vi "script user process vi.vi"(8 "error in":errorcluster, 10 "runtime class path in":path, 11 "Application in":refnum<vi>) -> (0 "error out":errorcluster)   [LabVIEW 2013]
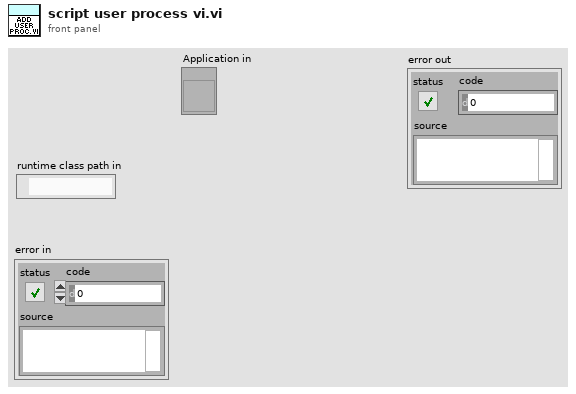
[diagram p1: front panel]
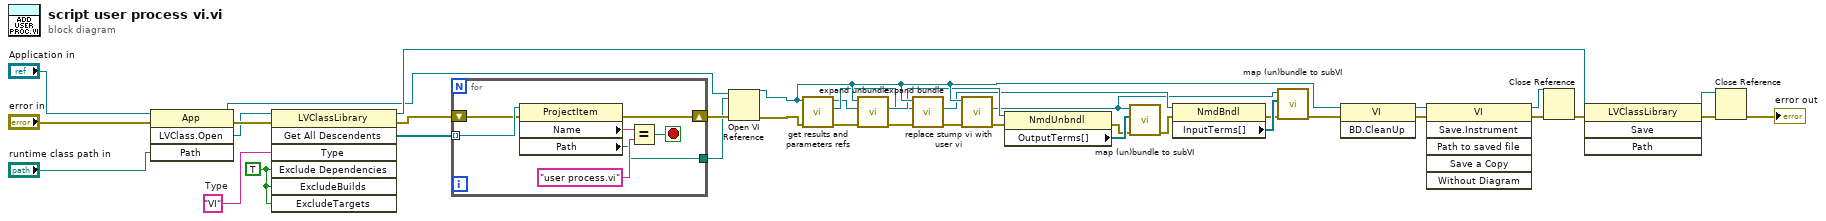
[diagram p0: block diagram]
diagram:
  w37 = TRUE
  w36 = "VI"  # Type
  n1 = invoke class="App" method="LVClass.Open"(reference="Application in", error in="error in", "Path"="runtime class path in") -> (reference out=w15:refnum<vi>, error out=w38:errorcluster, "LVClass.Open"=w16:refnum<vi>)  [unwired: 1 in, 1 out]
  n2 = invoke class="LVClassLibrary" method="Get All Descendents"(reference=w16, error in=w38, "Type"=w36, "Exclude Dependencies"=w37, "ExcludeBuilds"=w37, "ExcludeTargets"=w37) -> (reference out=w19:refnum<vi>, error out=w26:errorcluster, "All Descendents"=w33:refnum<vi>[])  [unwired: 1 in, 4 out]
  n3 = for {
    tunnel: w33 -> [w42] mode=indexing
    shift-right: [w40] -> w25
    shift-left: w26 -> [w41]
    tunnel: [w39] -> w24
    stop <- w43 stop-if-true
    n4 = property class="ProjectItem"(reference=w42, error in=w41) -> (error out=w40:errorcluster, "Name"=w45:string, "Path"=w39:path)  [unwired: 1 out]
    n5 = Equal?(x=w45, y="user process.vi") -> (x = y?=w43:bool)
  }
  n6 = Open VI Reference(application reference (local)=w15, vi path=w24, error in (no error)=w25) -> (vi reference=w22:refnum<vi>, error out=w23:errorcluster)  [unwired: 3 in]
  n7 = call "get results and parameters refs.vi"("error in"=w23, "VI in"=w22) -> ("error out"=w14:errorcluster, "Results from processing ref out"=w3:refnum<vi>, "Parameters to process ref out"=w2:refnum<vi>)  [unwired: 7 in]
  n8 = call "expand unbundle.vi"("error in"=w14, "Parameters to process ref in"=w2, "VI Refnum"=w22) -> ("error out"=w13:errorcluster, "unbundle ref out"=w11:refnum<vi>)  [unwired: 7 in]
  n9 = call "expand bundle.vi"("error in (no error)"=w13, "Results from processing ref in"=w3, "VI Refnum"=w22) -> ("error out"=w12:errorcluster, "Bundle ref out"=w7:refnum<vi>)  [unwired: 7 in]
  n10 = call "replace stump vi with user vi.vi"("error in (no error)"=w12, "VI in"=w22) -> ("error out"=w9:errorcluster, "subvi reference out"=w4:refnum<vi>)  [unwired: 8 in]
  n11 = property class="NmdUnbndl"(reference=w11, error in=w9) -> (error out=w8:errorcluster, "OutputTerms[]"=w10:refnum<vi>[])  [unwired: 1 out]
  n12 = call "map (un)bundle to subVI.vi"("error in (no error)"=w8, "Terms[]"=w10, "SubVI in"=w4) -> ("error out"=w1:errorcluster)  [unwired: 8 in]
  n13 = property class="NmdBndl"(reference=w7, error in=w1) -> (error out=w5:errorcluster, "InputTerms[]"=w6:refnum<vi>[])  [unwired: 1 out]
  n14 = call "map (un)bundle to subVI.vi"("error in (no error)"=w5, "Terms[]"=w6, "SubVI in"=w4) -> ("error out"=w32:errorcluster)  [unwired: 8 in]
  n15 = invoke class="VI" method="BD.CleanUp"(reference=w22, error in=w32) -> (reference out=w31:refnum<vi>, error out=w29:errorcluster)  [unwired: 1 in, 1 out]
  n16 = invoke class="VI" method="Save.Instrument"(reference=w31, error in=w29) -> (reference out=w30:refnum<vi>, error out=w28:errorcluster)  [unwired: 4 in, 4 out]
  n17 = Close Reference(reference=w30, error in (no error)=w28) -> (error out=w21:errorcluster)
  n18 = invoke class="LVClassLibrary" method="Save"(reference=w19, error in=w21) -> (reference out=w18:refnum<vi>, error out=w20:errorcluster)  [unwired: 2 in, 2 out]
  n19 = Close Reference(reference=w18, error in (no error)=w20) -> (error out=→"error out":errorcluster)
